vi "VMI_queue_set_up_arrays.vi"(3 "error in (no error)":errorcluster, 5 "Number of Queues":i32) -> (0 "error out":errorcluster, 1 "Stop":bool, 2 "Queue Array":T1[](array[typedef]))   [LabVIEW 2020]
doc: "This VI sets up the queues to allow images to be acquired at the same time as they are analysed. The number of queues sets up how many queues to create. The queues are produced as an array so can be any size"
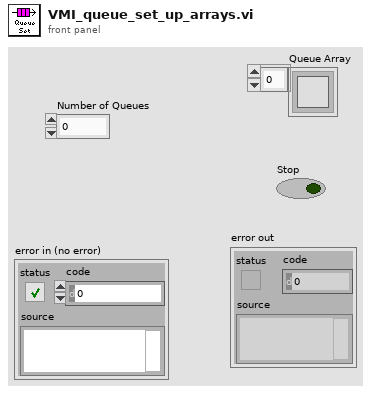
[diagram p1: front panel]
types:
  T1 = typedef "Queue RefNum" = refnum<k1>
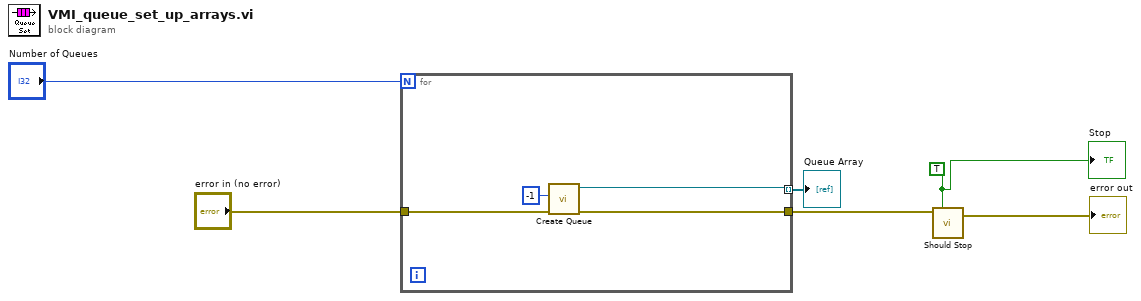
[diagram p0: block diagram]
diagram:
  w2 = TRUE ("Initialize")
  n1 = for {
    N: "Number of Queues" -> [_]
    tunnel: "error in (no error)" -> [w10]
    tunnel: [w9] -> w3
    tunnel: [w8] -> w4 mode=indexing
    n2 = call <vilib>:"Create Queue.vi"("error in (no error)"=w10, "size (unbounded)"=-1) -> ("error out"=w9:errorcluster, "queue out"=w8:T1)  [unwired: 3 in, 1 out]
  }
  "Queue Array" <- w4
  n3 = call "Should Stop.vi"("error in 1"=w3, "Initialize"=w2) -> ("error out"=→"error out":errorcluster)  [unwired: 3 in, 1 out]
  "Stop" <- w2
